vi "Replace_screw_and_nut.vi"(8 "Error In":errorcluster) -> (0 "Error Out":errorcluster)   [LabVIEW 2019]
uses:
  WSCbot_V3_Toolkit.lvlibp
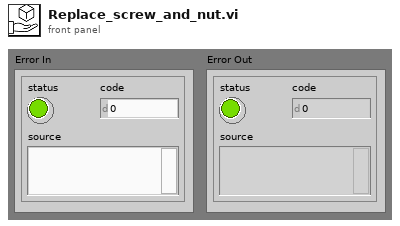
[diagram p1: front panel]
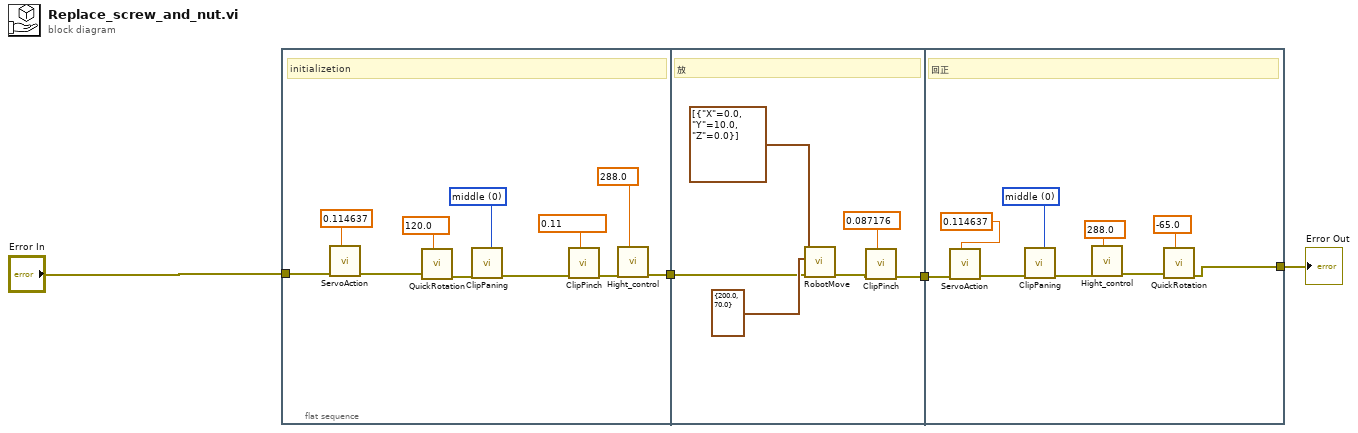
[diagram p0: block diagram]
diagram:
  n1 = flat-sequence {
    tunnel: "Error In" -> [w7]
    tunnel: [w8] -> w3
    tunnel: w3 -> [w19]
    tunnel: [w16] -> w2
    tunnel: w2 -> [w27]
    tunnel: [w22] -> w1
    frame #0 {
      w9 = 120.0 items=["Forward"=30.0, "Right"=120.0, "Left"=-65.0] ("螺桿面向")
      w10 = 288.0 items=["物料櫃第一格"=0.0, "物料櫃第二格"=85.0, "螺帽夾取高度"=128.0, "螺帽瞄準"=250.0, "最高"=288.0] ("螺桿高度")
      w12 = 0 items=["left"=2300, "right"=-3500, "lock screw"=1345, "lock_nut"=1167, "middle"=0] ("location")
      w14 = 0.114637 items=["up"=0.1095, "lock_up"=0.111528, "up_up"=0.114637, "down"=0.073446, "back"=0.037435, "back_back"=0.035] ("face_dir")
      w15 = 0.11 items=["pinch_up"=0.11, "release"=0.087176] ("pinch?")
      # "initializetion"
      n2 = call "ServoAction.vi"("face_dir"=w14, "Error In"=w7) -> ("Error Out"=w6:errorcluster)  [unwired: 9 in]
      n3 = call "QuickRotation.vi"("螺桿面向"=w9, "Error In"=w6) -> ("Error Out"=w13:errorcluster)  [unwired: 9 in]
      n4 = call "ClipPaning.vi"("Error In"=w13, "location"=w12) -> ("Error Out"=w5:errorcluster)  [unwired: 8 in]
      n5 = call "ClipPinch.vi"("pinch?"=w15, "Error In"=w5) -> ("Error Out"=w11:errorcluster)  [unwired: 9 in]
      n6 = call "Hight_control.vi"("螺桿高度"=w10, "Error In"=w11) -> ("Error Out"=w8:errorcluster)  [unwired: 9 in]
    }
    frame #1 {
      w17 = 0.087176 items=["pinch_up"=0.11, "release"=0.087176] ("pinch?")
      # "放"
      n7 = call "RobotMove.vi"("error in (no error)"=w19, "Speed/ACC"=cluster{dbl, dbl} {200.0, 70.0}, "XYZ"=cluster{"X":dbl, "Y":dbl, "Z":dbl}[] [{"X"=0.0, "Y"=10.0, "Z"=0.0}]) -> ("error out"=w18:errorcluster)  [unwired: 8 in]
      n8 = call "ClipPinch.vi"("pinch?"=w17, "Error In"=w18) -> ("Error Out"=w16:errorcluster)  [unwired: 9 in]
    }
    frame #2 {
      w30 = -65.0 items=["Forward"=30.0, "Right"=120.0, "Left"=-65.0] ("螺桿面向")
      w29 = 288.0 items=["物料櫃第一格"=0.0, "物料櫃第二格"=85.0, "螺帽夾取高度"=128.0, "螺帽瞄準"=250.0, "最高"=288.0] ("螺桿高度")
      w28 = 0 items=["left"=2300, "right"=-3500, "lock screw"=1345, "lock_nut"=1167, "middle"=0] ("location")
      w26 = 0.114637 items=["up"=0.1095, "lock_up"=0.111528, "up_up"=0.114637, "down"=0.073446, "back"=0.037435, "back_back"=0.035] ("face_dir")
      # "回正"
      n9 = call "ServoAction.vi"("face_dir"=w26, "Error In"=w27) -> ("Error Out"=w25:errorcluster)  [unwired: 9 in]
      n10 = call "ClipPaning.vi"("Error In"=w25, "location"=w28) -> ("Error Out"=w24:errorcluster)  [unwired: 8 in]
      n11 = call "Hight_control.vi"("螺桿高度"=w29, "Error In"=w24) -> ("Error Out"=w23:errorcluster)  [unwired: 9 in]
      n12 = call "QuickRotation.vi"("螺桿面向"=w30, "Error In"=w23) -> ("Error Out"=w22:errorcluster)  [unwired: 9 in]
    }
  }
  "Error Out" <- w1
